vi "File_BrowseDirectory.vi"(0 "DirPath":path, 1 "Treat LLB as directories?":bool, 5 "error in (no error)":errorcluster, 6 "Reset":bool) -> (12 "Ctts":T1[](array[typedef]), 14 "VIs":T1[](array[typedef]), 15 "Ctls":T1[](array[typedef]), 16 "VITs":T1[](array[typedef]), 17 "All":T1[](array[typedef]), 18 "directory names":string[](array[string]), 19 "error out":errorcluster)   [LabVIEW 2014]
uses:
  <resource>/Framework/Providers/Open_GDS/ClassProviders/Common/File/File_FileInfo.ctl
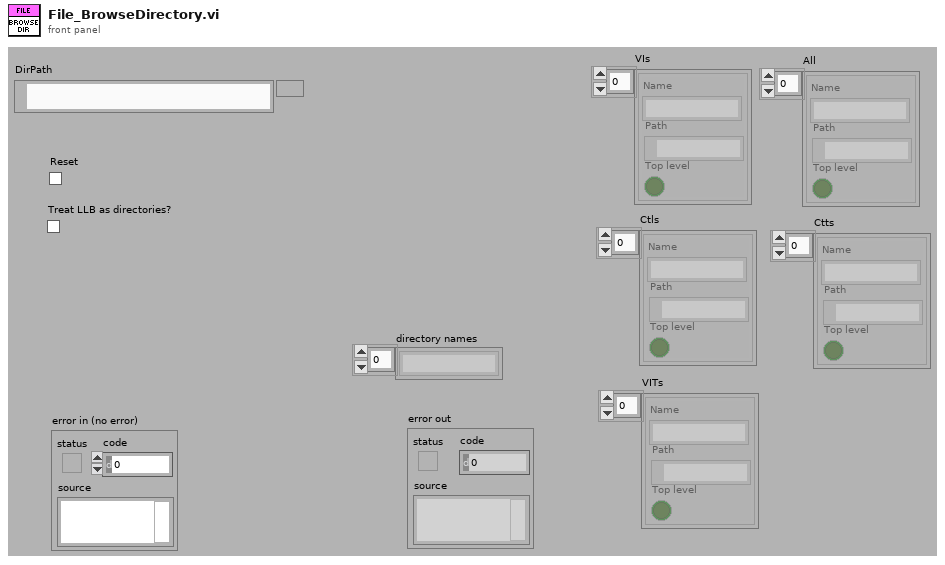
[diagram p1: front panel]
types:
  T1 = typedef "File_FileInfo.ctl" = cluster{"Name":string, "Path":path, "Top level":bool}
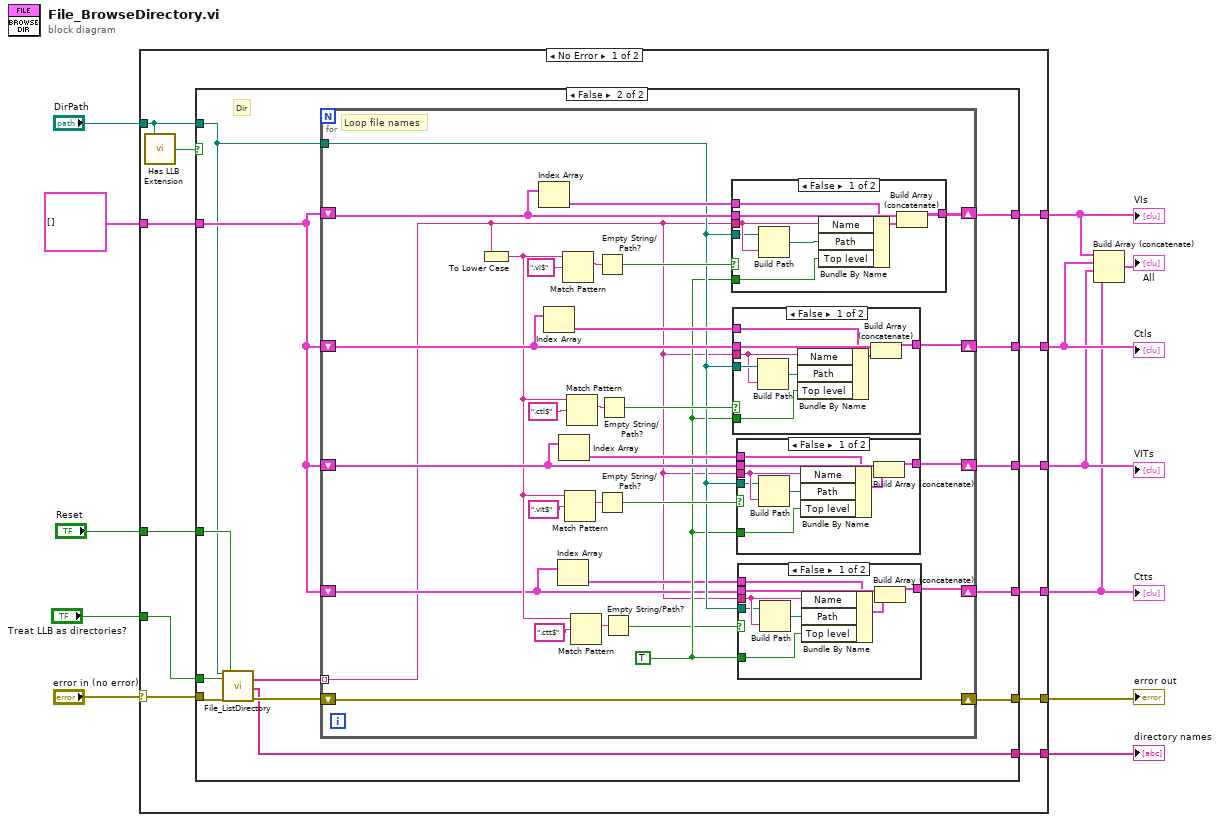
[diagram p0: block diagram]
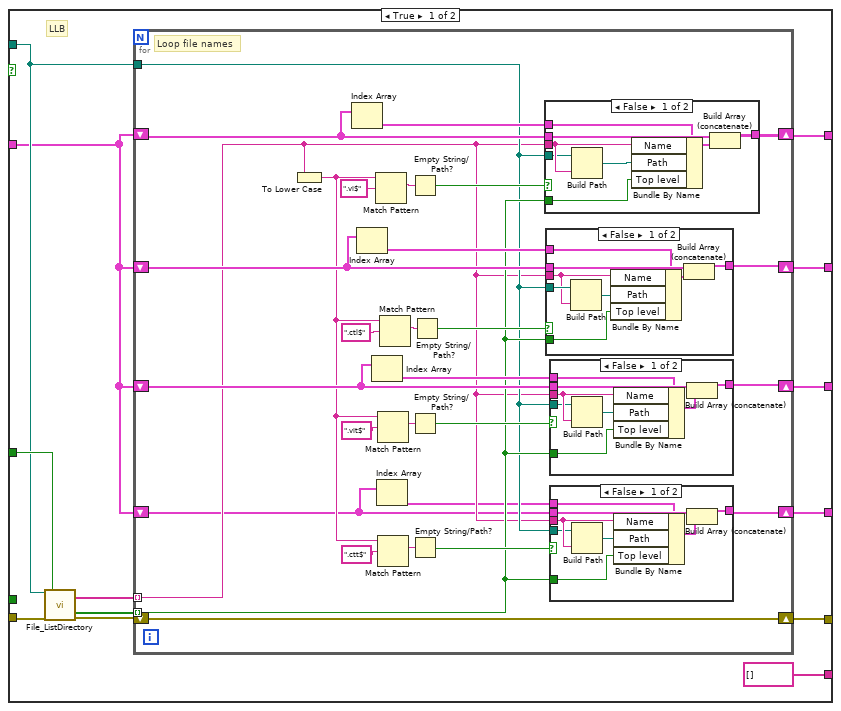
[diagram p2: hidden frame]
diagram:
  n1 = case shown="No Error" "error in (no error)" {
    selector: "error in (no error)" -> [w24 w183]
    tunnel: [w23 w183] -> w11
    tunnel: "DirPath" -> [w20 _]
    tunnel: [w21 w181] -> w6
    tunnel: [w22 string[] [] ("directory names")] -> w9
    tunnel: [w18 w181] -> w5
    tunnel: [w17 w181] -> w4
    tunnel: T1[] [] ("Array Constant") -> [w16 w181]
    tunnel: "Reset" -> [w15 _]
    tunnel: [w14 w181] -> w2
    tunnel: "Treat LLB as directories?" -> [w13 _]
    frame No Error {
      n2 = call <vilib>:"Has LLB Extension.vi"("path"=w20) -> ("path to VI library?"=w19:bool)
      n3 = case shown="False" w19 {
        tunnel: w24 -> [w31 w111]
        tunnel: [w36 w114] -> w23
        tunnel: [w37 w115] -> w21
        tunnel: [string[] [] ("directory names") w109] -> w22
        tunnel: w20 -> [w27 w105]
        tunnel: [w35 w113] -> w18
        tunnel: [w34 w112] -> w17
        tunnel: w16 -> [w25 w106]
        tunnel: w15 -> [w29 w107]
        tunnel: [w26 w104] -> w14
        tunnel: w13 -> [_ w103]
        frame True {
          # "LLB"
          n4 = call <resource>:"File_ListDirectory.vi"("Directory Path"=w27, "error in (no error)"=w31, "Reset"=w29) -> ("File names"=w30:string[], "Top level"=w28:bool[], "error out"=w32:errorcluster)  [unwired: 2 in, 12 out]
          n5 = for {
            shift-right: [w65] -> w37
            shift-left: w25 -> [w66]
            shift-right: [w48] -> w36
            shift-left: w32 -> [w48]
            shift-right: [w64] -> w35
            shift-left: w25 -> [w52]
            shift-right: [w63] -> w34
            shift-left: w25 -> [w50]
            tunnel: w27 -> [w41]
            tunnel: w30 -> [w40] mode=indexing
            tunnel: w28 -> [w42] mode=indexing
            shift-right: [w45] -> w26
            shift-left: w25 -> [w39]
            # "Loop file names"
            n6 = To Lower Case(string=w40) -> (all lower case string=w44:string)
            n7 = Index Array(array=w66) -> (element=w53:T1)  [unwired: 1 in]
            n8 = Index Array(array=w52) -> (element=w51:T1)  [unwired: 1 in]
            n9 = Index Array(array=w50) -> (element=w49:T1)  [unwired: 1 in]
            n10 = Match Pattern(string=w44, regular expression=".vi$") -> (match substring=w62:string)  [unwired: 4 out]
            n11 = Index Array(array=w39) -> (element=w38:T1)  [unwired: 1 in]
            n12 = Match Pattern(string=w44, regular expression=".vit$") -> (match substring=w60:string)  [unwired: 4 out]
            n13 = Match Pattern(string=w44, regular expression=".ctt$") -> (match substring=w46:string)  [unwired: 4 out]
            n14 = Match Pattern(string=w44, regular expression=".ctl$") -> (match substring=w61:string)  [unwired: 4 out]
            n15 = Empty String/Path?(string/path=w62) -> (empty?=w57:bool)
            n16 = Empty String/Path?(string/path=w60) -> (empty?=w59:bool)
            n17 = Empty String/Path?(string/path=w46) -> (empty?=w43:bool)
            n18 = Empty String/Path?(string/path=w61) -> (empty?=w58:bool)
            n19 = case shown="False" w57 {
              tunnel: w40 -> [w96 _]
              tunnel: w66 -> [w101 w102]
              tunnel: [w100 w102] -> w65
              tunnel: w53 -> [w99 _]
              tunnel: w42 -> [w95 _]
              tunnel: w41 -> [w94 _]
              frame False {
                n20 = Build Path(base path=w94, name or relative path=w96) -> (appended path=w97:path)
                n21 = Bundle By Name(cluster=w99, "Name"=w96, "Path"=w97, "Top level"=w95) -> (w98:T1)
                n22 = Build Array (concatenate)(w101, w98) -> (w100:T1[])
              }
              frame True {
              }
            }
            n23 = case shown="False" w58 {
              tunnel: w40 -> [w86 _]
              tunnel: w52 -> [w92 w93]
              tunnel: [w91 w93] -> w64
              tunnel: w51 -> [w89 _]
              tunnel: w41 -> [w87 _]
              tunnel: w42 -> [w85 _]
              frame False {
                n24 = Build Path(base path=w87, name or relative path=w86) -> (appended path=w88:path)
                n25 = Bundle By Name(cluster=w89, "Name"=w86, "Path"=w88, "Top level"=w85) -> (w90:T1)
                n26 = Build Array (concatenate)(w92, w90) -> (w91:T1[])
              }
              frame True {
              }
            }
            n27 = case shown="False" w59 {
              tunnel: w40 -> [w78 _]
              tunnel: w50 -> [w83 w84]
              tunnel: [w82 w84] -> w63
              tunnel: w49 -> [w80 _]
              tunnel: w41 -> [w77 _]
              tunnel: w42 -> [w76 _]
              frame False {
                n28 = Build Path(base path=w77, name or relative path=w78) -> (appended path=w79:path)
                n29 = Bundle By Name(cluster=w80, "Name"=w78, "Path"=w79, "Top level"=w76) -> (w81:T1)
                n30 = Build Array (concatenate)(w83, w81) -> (w82:T1[])
              }
              frame True {
              }
            }
            n31 = case shown="False" w43 {
              tunnel: w40 -> [w69 _]
              tunnel: w39 -> [w74 w75]
              tunnel: [w73 w75] -> w45
              tunnel: w38 -> [w71 _]
              tunnel: w41 -> [w68 _]
              tunnel: w42 -> [w67 _]
              frame False {
                n32 = Build Path(base path=w68, name or relative path=w69) -> (appended path=w70:path)
                n33 = Bundle By Name(cluster=w71, "Name"=w69, "Path"=w70, "Top level"=w67) -> (w72:T1)
                n34 = Build Array (concatenate)(w74, w72) -> (w73:T1[])
              }
              frame True {
              }
            }
          }
        }
        frame False {
          # "Dir"
          n35 = call <resource>:"File_ListDirectory.vi"("Directory Path"=w105, "Treat LLB as directories?"=w103, "error in (no error)"=w111, "Reset"=w107) -> ("File names"=w108:string[], "Directory names"=w109:string[], "error out"=w110:errorcluster)  [unwired: 1 in, 12 out]
          n36 = for {
            shift-right: [w143] -> w115
            shift-left: w106 -> [w144]
            shift-right: [w126] -> w114
            shift-left: w110 -> [w126]
            shift-right: [w142] -> w113
            shift-left: w106 -> [w130]
            shift-right: [w141] -> w112
            shift-left: w106 -> [w128]
            tunnel: w105 -> [w122]
            tunnel: w108 -> [w116] mode=indexing
            shift-right: [w125] -> w104
            shift-left: w106 -> [w117]
            w121 = TRUE
            # "Loop file names"
            n37 = To Lower Case(string=w116) -> (all lower case string=w119:string)
            n38 = Index Array(array=w144) -> (element=w131:T1)  [unwired: 1 in]
            n39 = Index Array(array=w130) -> (element=w129:T1)  [unwired: 1 in]
            n40 = Index Array(array=w117) -> (element=w118:T1)  [unwired: 1 in]
            n41 = Index Array(array=w128) -> (element=w127:T1)  [unwired: 1 in]
            n42 = Match Pattern(string=w119, regular expression=".vi$") -> (match substring=w140:string)  [unwired: 4 out]
            n43 = Match Pattern(string=w119, regular expression=".vit$") -> (match substring=w138:string)  [unwired: 4 out]
            n44 = Match Pattern(string=w119, regular expression=".ctl$") -> (match substring=w139:string)  [unwired: 4 out]
            n45 = Match Pattern(string=w119, regular expression=".ctt$") -> (match substring=w123:string)  [unwired: 4 out]
            n46 = Empty String/Path?(string/path=w140) -> (empty?=w135:bool)
            n47 = Empty String/Path?(string/path=w138) -> (empty?=w137:bool)
            n48 = Empty String/Path?(string/path=w139) -> (empty?=w136:bool)
            n49 = Empty String/Path?(string/path=w123) -> (empty?=w120:bool)
            n50 = case shown="False" w135 {
              tunnel: w116 -> [w174 _]
              tunnel: w144 -> [w179 w180]
              tunnel: [w178 w180] -> w143
              tunnel: w131 -> [w177 _]
              tunnel: w121 -> [w173 _]
              tunnel: w122 -> [w172 _]
              frame False {
                n51 = Build Path(base path=w172, name or relative path=w174) -> (appended path=w175:path)
                n52 = Bundle By Name(cluster=w177, "Name"=w174, "Path"=w175, "Top level"=w173) -> (w176:T1)
                n53 = Build Array (concatenate)(w179, w176) -> (w178:T1[])
              }
              frame True {
              }
            }
            n54 = case shown="False" w136 {
              tunnel: w116 -> [w164 _]
              tunnel: w130 -> [w170 w171]
              tunnel: [w169 w171] -> w142
              tunnel: w129 -> [w167 _]
              tunnel: w122 -> [w165 _]
              tunnel: w121 -> [w163 _]
              frame False {
                n55 = Build Path(base path=w165, name or relative path=w164) -> (appended path=w166:path)
                n56 = Bundle By Name(cluster=w167, "Name"=w164, "Path"=w166, "Top level"=w163) -> (w168:T1)
                n57 = Build Array (concatenate)(w170, w168) -> (w169:T1[])
              }
              frame True {
              }
            }
            n58 = case shown="False" w137 {
              tunnel: w116 -> [w156 _]
              tunnel: w128 -> [w161 w162]
              tunnel: [w160 w162] -> w141
              tunnel: w127 -> [w158 _]
              tunnel: w122 -> [w155 _]
              tunnel: w121 -> [w154 _]
              frame False {
                n59 = Build Path(base path=w155, name or relative path=w156) -> (appended path=w157:path)
                n60 = Bundle By Name(cluster=w158, "Name"=w156, "Path"=w157, "Top level"=w154) -> (w159:T1)
                n61 = Build Array (concatenate)(w161, w159) -> (w160:T1[])
              }
              frame True {
              }
            }
            n62 = case shown="False" w120 {
              tunnel: w116 -> [w147 _]
              tunnel: w117 -> [w152 w153]
              tunnel: [w151 w153] -> w125
              tunnel: w118 -> [w149 _]
              tunnel: w122 -> [w146 _]
              tunnel: w121 -> [w145 _]
              frame False {
                n63 = Build Path(base path=w146, name or relative path=w147) -> (appended path=w148:path)
                n64 = Bundle By Name(cluster=w149, "Name"=w147, "Path"=w148, "Top level"=w145) -> (w150:T1)
                n65 = Build Array (concatenate)(w152, w150) -> (w151:T1[])
              }
              frame True {
              }
            }
          }
        }
      }
    }
    frame Error {
    }
  }
  "error out" <- w11
  "directory names" <- w9
  "VITs" <- w4
  "Ctls" <- w5
  "VIs" <- w6
  "Ctts" <- w2
  n66 = Build Array (concatenate)(w6, w5, w4, w2) -> (→"All":T1[])
